vi "GMLAN SecurityAccess.vi"   [LabVIEW 2013, in "GMLAN.lvlib"]
uses:
  GMLAN.lvlib
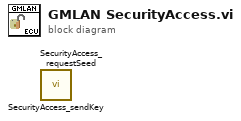
[diagram p0: block diagram]
diagram:
  n1 = call "SecurityAccess_sendKey.vi"() -> ()  [unwired: 9 in, 3 out]
  n2 = call "SecurityAccess_requestSeed.vi"() -> ()  [unwired: 8 in, 4 out]
